vi "Probabilities.vi"(9 "Final state? (T)":bool=TRUE, 11 "Circuit cluster":T1) -> (3 "Probabilities":dbl[](array[numeric]))   [LabVIEW 2016]
uses:
  TypeDefs/Circuit Cluster.ctl
  Classes/GateAbst/GateAbst.lvclass
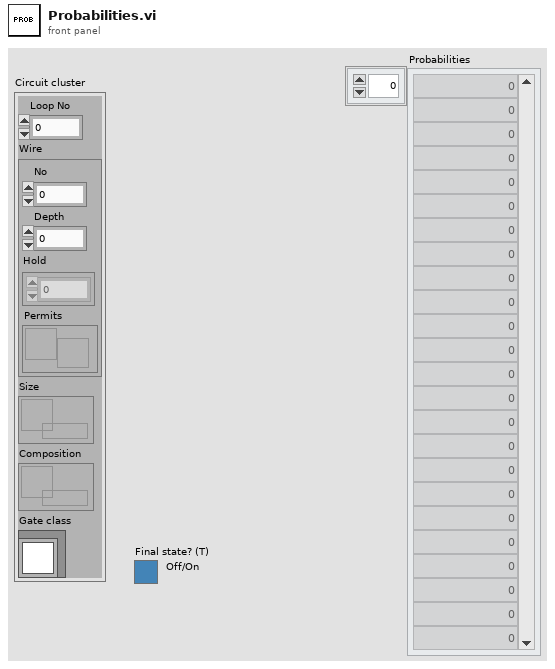
[diagram p1: front panel]
types:
  T1 = typedef "Circuit Cluster.ctl" = cluster{"Loop No":i32, "Wire":cluster{"No":i32, "Depth":i32, "Hold":i32[][], "Permits":refnum<notifier>}, "Size":refnum<queue>, "Composition":refnum<queue>, "Gate class":refnum<class "GateAbst.lvclass">}
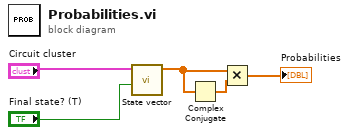
[diagram p0: block diagram]
diagram:
  n1 = call "State vector.vi"("Final state? (T)"="Final state? (T)", "Circuit cluster"="Circuit cluster") -> ("State vector"=w2:cdb[])  [unwired: 9 in]
  n2 = Complex Conjugate(1:w2) -> (0:w5:cdb[])
  n3 = Multiply(x=w2, y=w5) -> (x*y=→"Probabilities":cdb[])
